vi "FA_AgentConfig_GetDebugStatus.vi"(8 "Error In":errorcluster) -> (0 "Error Out":errorcluster, 2 "DebugStatus":bool)   [LabVIEW 2014, in "FA_AgentConfig.lvlib"]
doc: "Returns the key value for DebugStatus in FA_Config.ini"
uses:
  FA_AgentConfig.lvlib
  FA_LocalStore API/source/VI Source/FA_LSSpecialTypes.ctl
  FA_LocalStore API/source/VI Source/FA_LocalStore.lvlib
  FA_NativeTypes API/source/VI Source/FA_NativeTypes.lvlib
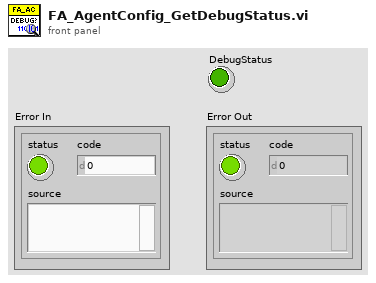
[diagram p1: front panel]
types:
  T1 = typedef "FA_LocalStore.lvlib/FA_LSSpecialTypes.ctl" = string
  T2 = typedef "FA_NativeTypes.lvlib/FA_Config.ctl" = cluster{"Id":string, "Name":T1, "Parameter":cluster{"Name":string, "Value":string}[], "Account":string, "CreateDate":string, "LastModified":string}
  T3 = typedef "FA_AgentConfig.lvlib/FA_AgentConfig.ctl" = cluster{"x-ni-client-id":string, "x-ni-apikey":string, "CloudLookupTime":u32, "Debug":bool, "DeviceName":string}
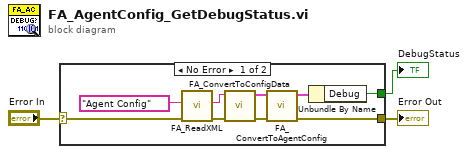
[diagram p0: block diagram]
diagram:
  n1 = case shown="No Error" "Error In" {
    selector: "Error In" -> [w11 w13]
    tunnel: [w7 w13] -> w2
    tunnel: [w4 _] -> w1
    frame No Error {
      n2 = call "FA_ReadXML.vi"("Error In"=w11, "Special Type"=T1 "Agent Config") -> ("Error Out"=w10:errorcluster, "XML String"=w9:string)  [unwired: 6 in]
      n3 = call "FA_ConvertToConfigData.vi"("Error In"=w10, "XML String"=w9) -> ("Error Out"=w8:errorcluster, "ConfigData"=w6:T2)  [unwired: 8 in]
      n4 = call "FA_ConvertToAgentConfig.vi"("Error In"=w8, "Config"=w6) -> ("Error Out"=w7:errorcluster, "AgentConfig"=w5:T3)  [unwired: 8 in]
      n5 = Unbundle By Name(w5) -> ("Debug"=w4:bool)
    }
    frame Error {
    }
  }
  "Error Out" <- w2
  "DebugStatus" <- w1
